vi "ValveControlHandler.vi"(1 "Override Control Outputs":bool[](array[boolean]), 3 "Solenoid NC/NO":bool[](array[boolean]), 4 "Relay NO/NC":bool[](array[boolean]), 5 "Manual Abort":bool, 6 "Solenoid Supply Voltage":dbl, 7 "Manual Override":bool, 8 "Valve Diagnostics":bool, 9 "Control System Outputs":bool[](array[boolean]), 10 "Abort":bool) -> (0 "Solenoid Control":bool[](array[boolean]), 2 "Valve Diagnostics":bool[](array[boolean]))   [LabVIEW 2021]
panel:
  # "Manual Override"
  # "Procedural Control System"
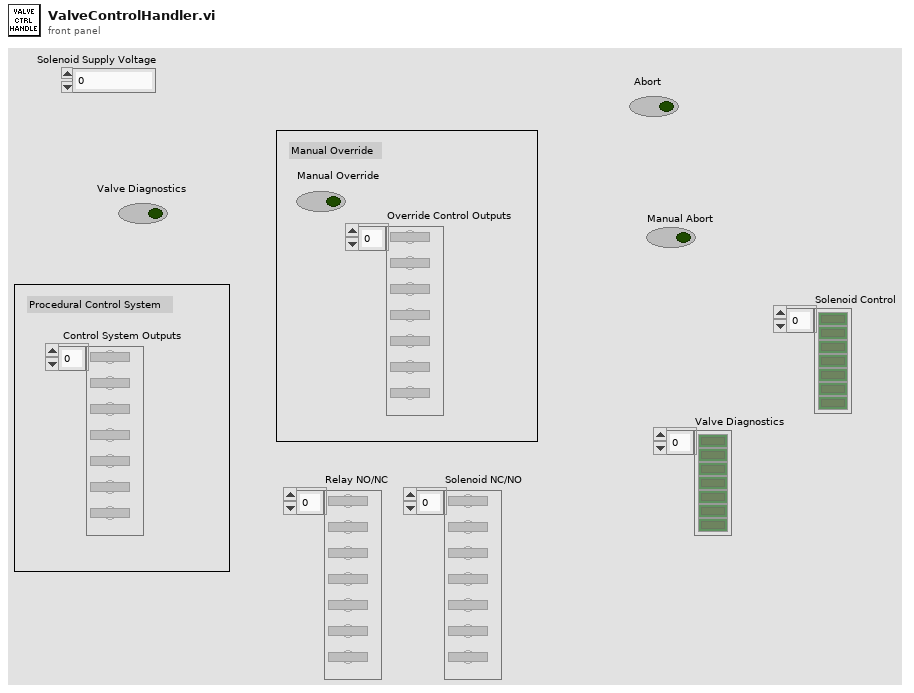
[diagram p1: front panel]
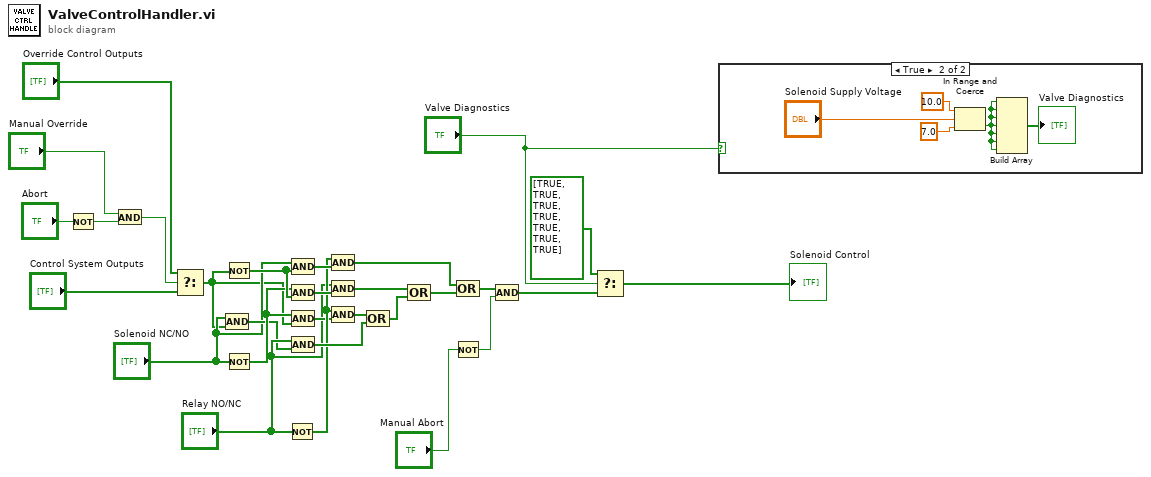
[diagram p0: block diagram]
diagram:
  n1 = Not(x="Abort") -> (.not. x?=w27:bool)
  n2 = And(x="Manual Override", y=w27) -> (x .and. y?=w26:bool)
  n3 = Select(t="Override Control Outputs", s=w26, f="Control System Outputs") -> (s? t:f=w5:bool[])
  n4 = Not(x=w5) -> (.not. x?=w22:bool[])
  n5 = Not(x="Solenoid NC/NO") -> (.not. x?=w14:bool[])
  n6 = Compound Arithmetic op=AND("Solenoid NC/NO", w5) -> (w12:bool[])
  n7 = Not(x="Relay NO/NC") -> (.not. x?=w16:bool[])
  n8 = Compound Arithmetic op=AND("Solenoid NC/NO", w22) -> (w25:bool[])
  n9 = Compound Arithmetic op=AND(w14, w22) -> (w23:bool[])
  n10 = Compound Arithmetic op=AND(w14, w5) -> (w15:bool[])
  n11 = Compound Arithmetic op=AND("Relay NO/NC", w12) -> (w17:bool[])
  n12 = Compound Arithmetic op=AND(w16, w25) -> (w24:bool[])
  n13 = Compound Arithmetic op=AND("Relay NO/NC", w23) -> (w20:bool[])
  n14 = Compound Arithmetic op=AND(w16, w15) -> (w18:bool[])
  n15 = Compound Arithmetic op=OR(w18, w17) -> (w19:bool[])
  n16 = Compound Arithmetic op=OR(w20, w19) -> (w21:bool[])
  n17 = Not(x="Manual Abort") -> (.not. x?=w9:bool)
  n18 = Compound Arithmetic op=OR(w24, w21) -> (w10:bool[])
  n19 = Compound Arithmetic op=AND(w10, w9) -> (w2:bool[])
  n20 = Select(t=bool[] [TRUE, TRUE, TRUE, TRUE, TRUE, TRUE, TRUE] ("Valve Diagnostics Outputs"), s="Valve Diagnostics", f=w2) -> (s? t:f=→"Solenoid Control":bool[])
  n21 = case shown="True" "Valve Diagnostics" {
    frame False {
    }
    frame True {
      n22 = In Range and Coerce(upper limit=10.0, x="Solenoid Supply Voltage", lower limit=7.0) -> (In Range?=w34:bool)  [unwired: 1 out]
      n23 = Build Array(w34, w34, w34, w34, w34, w34, w34) -> (→"Valve Diagnostics":bool[])
    }
  }
